vi "Sys A TXRX Host.vi"() -> ()   [LabVIEW 2019]
uses:
  SubVIs/mmWave HW Control/HW TXRX resources cluster.ctl
  <instrlib>/niMmWave/ni3610 and ni3630/controls/public/Board Information.ctl
  <instrlib>/niMmWave/ni3610 and ni3630/private/mm/Typedefs/PID.ctl
  <instrlib>/niMmWave/ni3610 and ni3630/controls/private/Board Hardware Revision.ctl
  SubVIs/mmWave HW Control/HW TXRX RF config cluster.ctl
  SubVIs/mmWave HW Control/HW Timing module config cluster.ctl
  SubVIs/mmWave HW Control/RX acquisition config.ctl
  SubVIs/Low-level/TypeDefs/TX trigger config.ctl
  FPGA/SubVIs/Utility/FPGA driver trigger source.ctl
  FPGA/SubVIs/Utility/FPGA driver trigger destination.ctl
  SubVIs/Low-level/TypeDefs/Front End Configuration.ctl
  SubVIs/Low-level/TypeDefs/Channel Configuration.ctl
  <instrlib>/niMmWave/ni3620/Config/v1/Host/Public/Typedefs/mmWave Port.ctl
  SubVIs/mmWave HW Control/HW state enum.ctl
  <vilib>/Utility/error.llb/DialogType.ctl
  SubVIs/mmWave HW Control/Message and Data cluster.ctl
  SubVIs/Low-level/TypeDefs/Hardware Configuration.ctl
  SubVIs/Low-level/TypeDefs/Direction.ctl
  SubVIs/Low-level/TypeDefs/Resources.ctl
  <vilib>/userdefined/High Color/nirio_resource_hc.ctl
  SubVIs/mmWave HW Control/TXRX generation acquisition config.ctl
  <vilib>/Analysis/4window.llb/windowTd.ctl
  <vilib>/measure/maspectr.llb/Power Spectrum and PSD Export Mode.ctl
  60642c00-3acc-4c81-b220-e8d2fc82becf.vi
  <vilib>/Analysis/2dsp.llb/1D Convolution (CDB).vi
  <vilib>/measure/maspectr.llb/FFT Power Spectrum and PSD for 1 Chan.vi
  Intertarget communication/NS master_class/NS master.lvclass
  SubVIs/mmWave HW Control/mmWave HW Control.lvlib
  <vilib>/Analysis/NI_AALPro.lvlib
  <instrlib>/niMmWave/ni3610 and ni3630/ni3610_and_ni3630_Driver_Lib.lvlib
  <instrlib>/niMmWave/ni3620/Config/v1/Host/niMmWave Config v1 Host.lvlib
  FPGA/SubVIs/Utility/FPGA Utility.lvlib
  <vilib>/measure/NI_MAPro.lvlib
  SubVIs/FPGA sequener API/FPGA sequencer API.lvlib
panel:
  out "burst memo":enum16{"DRAM", "BRAM"}(ring)
  out "last wr addr":u32
  in  "txrx.trigger":bool
  in  "stop scirpt":bool
  in  "Data view tab":T1(tab)
  out "Waveform plot":sgl[][](graph)
  in  "Averaging control":bool
  out "Power spectrum":cluster{"f0":dbl, "df":dbl, "magnitude":dbl[]}(graph)
  in  "averaging parameters":T2={"averaging mode"=enum."Peak hold", "weighting mode"=enum."Exponential", "number of averages"=50} {"number of averages" min=1}
  out "RXB-TXA stat":cluster{"Count":i32, "Mean":dbl, "Std":dbl} {"Std" format="%#_6p"; "Mean" format="%#_6p"}
  in  "Reset statistics":bool
  out "Time histogram":T3(graph) caption="XY Graph - Dark"
  out "RXA-TXA stat":cluster{"Count":i32, "Mean":dbl, "Std":dbl} {"Std" format="%#_6p"; "Mean" format="%#_6p"}
  out "RXB-RXA stat":cluster{"Count":i32, "Mean":dbl, "Std":dbl} {"Std" format="%#_6p"; "Mean" format="%#_6p"}
  in  "Repeat script":i32
  in  "Script.start":bool
  in  "Script":string="A \"hw.init\"\nB \"hw.reinit\" D 45000\nA \"txrx.start\" D500\nB \"rx.start\" D2000\nA \"txrx.trigger\" D200 R100\nA \"txrx.stop\"\nB \"rx.stop\""
  out "Last executed command":T4={"System"="", "Command"="", "Delay"=0, "Repeat"=1}
  out "script ctr":i32
  out "step ctr":i32
  out "R ctr":i32
  out "TX IQ":cdb[](array[numeric])
  out "Samples":u32
  out "coerced device configuration [channel]":T5[](array[typedef])=[{"port select"=enum."Loopback", "Rx hardware configuration"={"gain (dB)"=15.0, "frequency (Hz)"=12000000000.0, "mmWave adapter"="None", "adapter active port"=""}, "Tx hardware configuration"={"gain (dB)"=-15.0, "frequency (Hz)"=12000000000.0, "mmWave adapter"="None", "adapter active port"=""}}] {"Tx hardware configuration"."frequency (Hz)" format="%#_6p"; "Rx hardware configuration"."frequency (Hz)" format="%#_6p"}
  out "RXB-TX delay":dbl format="%#.3ps"
  out "Tx information":T8={"product code"=30638, "hardware revision"=enum."B", "serial number"="MTX1008\u0000"} {"product code" items=["PXIe-3610 I/Q Generator"=30638, "PXIe-3630 I/Q Digitizer"=30639]}
  in  "txrx.stop":bool
  out "Elements Remaining":u32
  in  "Stop Button":bool
  out "error out":T11
  in  "Tab Control":T12(tab)
  in  "HW.TXRX resources":T13={"TX_DAC"="Tx_DAC", "TX_FPGA"="Tx_FPGA", "IF"="IF_mod_demod", "RX_ADC"="Rx_ADC", "RX_FPGA"="Rx_FPGA"} caption="Reciever resources"
  in  "RF config":T14={"TX.Frequency"=0.0, "TX.Gain"=-10.0, "TX.mmWave adapter"="mmWave1/0", "RX.Frequency"=76000000000.0, "RX.Gain"=0.0, "RX.mmWave adapter"="mmWave0/0"} {"RX.Frequency" format="%#_6pHz"; "RX.Gain" format="%#_6fdb"; "TX.Frequency" format="%#_6pHz"; "TX.Gain" format="%#_6pHz"}
  in  "hw.init":bool
  in  "TX trigger options":T15
  in  "hw.conf trig":bool
  in  "HW.trig share config":T18={"mode"=enum."Export trig", "Timing module"="Dev1", "PXI line"="PXI_Trig1", "Module terminal"="PFI2"}
  in  "RX trigger options":T15={"delay"=8e-07, "trig source"=enum."Use Tclk", "PXI src"=0, "export"=enum."Synced trig", "PXI dest"=1} {"delay" format="%.0p"}
  in  "Repeat":bool
  in  "IQ waveform":string(combo)
  out "IQ preview":waveform(dbl)[](graph)
  out "Status":string
  in  "SysB.stop rx":bool
  in  "SysB.start rx":bool
  in  "SysB.hw reinit":bool
  in  "SysB.Connect":bool
  in  "Sys B IP address":string="192.168.40.171"
  in  "Plot":bool=TRUE
  out "dt":dbl=3.2552083333333335e-10 format="%#_6ps"
  in  "RX.read config":T19={"Samples"=320000}
  in  "txrx.start":bool
  out "Rx information":T8={"product code"=30639, "hardware revision"=enum."Unknown", "serial number"=""} {"product code" items=["PXIe-3610 I/Q Generator"=30638, "PXIe-3630 I/Q Digitizer"=30639]}
  out "RXA-TX delay":dbl format="%#.3ps"
  out "compensated max":i32
  out "max corr index":i32
  out "State":string
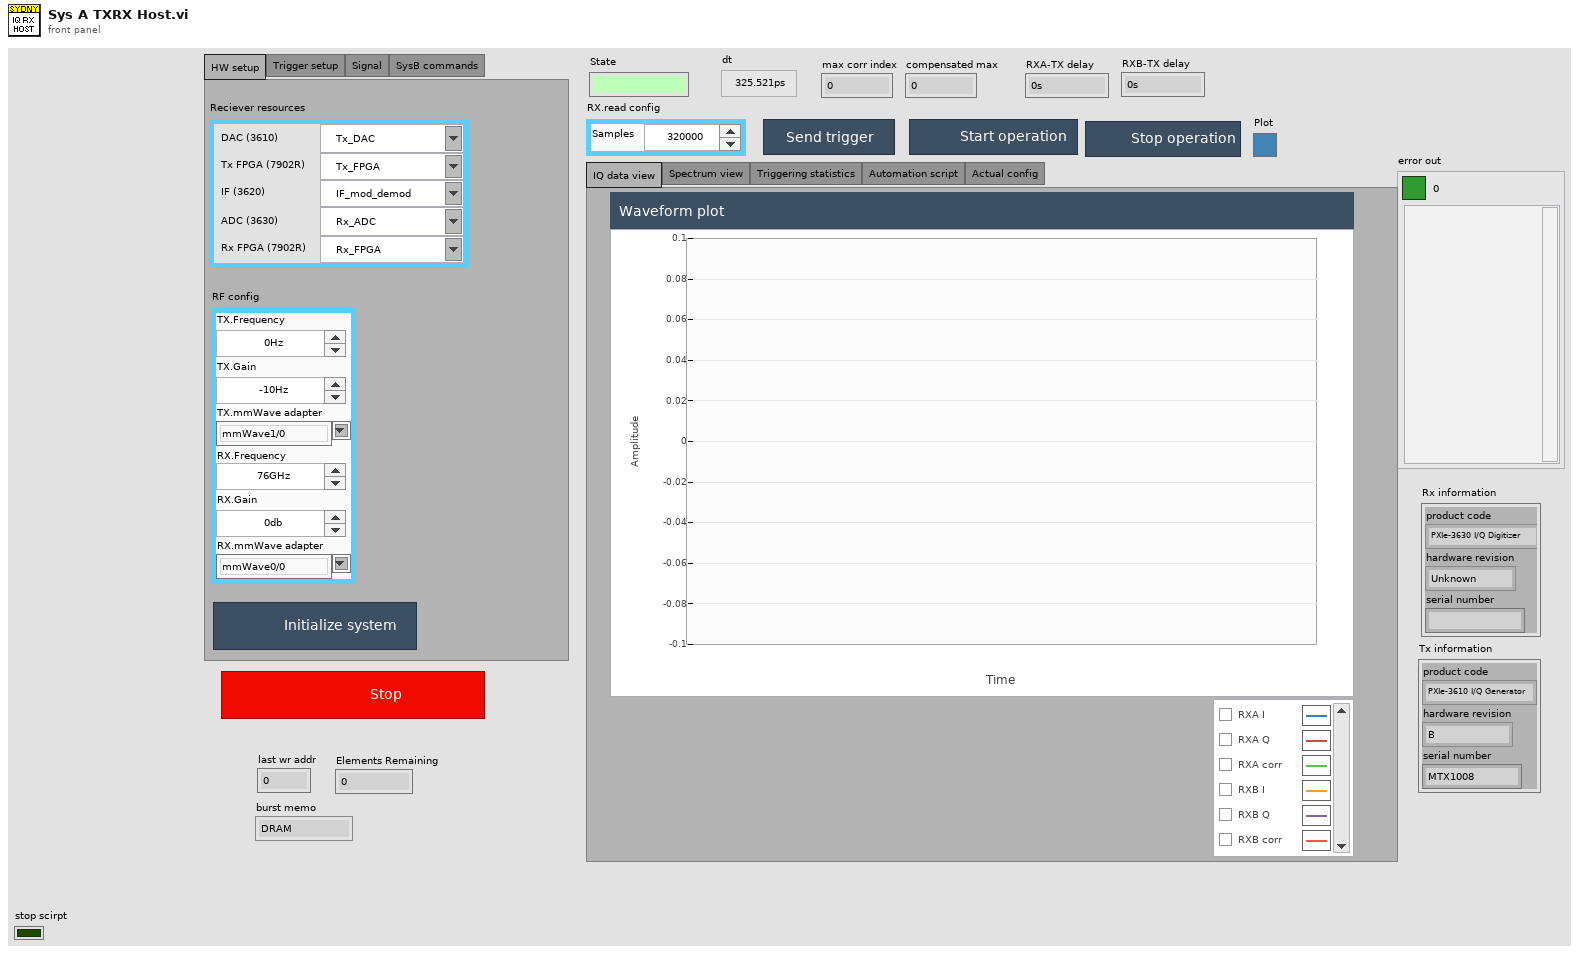
[diagram p1: front panel]
types:
  T1 = enum32{"IQ data view", "Spectrum view", "Triggering statistics", "Automation script", "Actual config"}
  T2 = cluster{"averaging mode":enum16{"No averaging", "Vector averaging", "RMS averaging", "Peak hold"}, "weighting mode":enum16{"Linear", "Exponential"}, "number of averages":u32}
  T3 = cluster{"X Values":dbl[], "Histogram: h(x)":i32[]}[]
  T4 = cluster{"System":string, "Command":string, "Delay":i32, "Repeat":i32}
  T5 = typedef "Front End Configuration.ctl" = cluster{"port select":enum16{"IF Port", "Loopback", "Sync Port"}, "Rx hardware configuration":T6, "Tx hardware configuration":T6}
  T6 = typedef "Channel Configuration.ctl" = cluster{"gain (dB)":dbl, "frequency (Hz)":dbl, "mmWave adapter":string, "adapter active port":T7}
  T7 = typedef "niMmWave Config v1 Host.lvlib/mmWave Port.ctl" = string
  T8 = typedef "Board Information.ctl" = cluster{"product code":T9, "hardware revision":T10, "serial number":string}
  T9 = typedef "ni3610_and_ni3630_Driver_Lib.lvlib/PID.ctl" = u16
  T10 = typedef "Board Hardware Revision.ctl" = enum16{"Unknown", "A", "B", "C", "D", "E", "F", "G", "H"}
  T11 = cluster{"Boolean Round":bool, "code":i32, "source":string}
  T12 = enum32{"HW setup", "Trigger setup", "Signal", "SysB commands"}
  T13 = typedef "mmWave HW Control.lvlib/HW TXRX resources cluster.ctl" = cluster{"TX_DAC":refnum<visa-resource-name>, "TX_FPGA":tag, "IF":tag, "RX_ADC":refnum<visa-resource-name>, "RX_FPGA":tag}
  T14 = typedef "mmWave HW Control.lvlib/HW TXRX RF config cluster.ctl" = cluster{"TX.Frequency":dbl, "TX.Gain":dbl, "TX.mmWave adapter":string, "RX.Frequency":dbl, "RX.Gain":dbl, "RX.mmWave adapter":string}
  T15 = typedef "TX trigger config.ctl" = cluster{"delay":dbl, "trig source":T16, "PXI src":i32, "export":T17, "PXI dest":i32}
  T16 = typedef "FPGA Utility.lvlib/FPGA driver trigger source.ctl" = enum16{"Use Tclk", "PXI_Trig", "Aurora RX trig"}
  T17 = typedef "FPGA Utility.lvlib/FPGA driver trigger destination.ctl" = enum16{"None", "Source trig", "Synced trig", "Delayed sync"}
  T18 = typedef "mmWave HW Control.lvlib/HW Timing module config cluster.ctl" = cluster{"mode":enum16{"None", "Export trig", "Import trig"}, "Timing module":tag, "PXI line":string, "Module terminal":string}
  T19 = typedef "mmWave HW Control.lvlib/RX acquisition config.ctl" = cluster{"Samples":u32}
  T20 = typedef "mmWave HW Control.lvlib/HW state enum.ctl" = enum16{"idle", "configuration", "running", "exit"}
  T21 = typedef "mmWave HW Control.lvlib/Message and Data cluster.ctl" = cluster{"message":string, "data":variant}
  T22 = typedef "Resources.ctl" = cluster{"7902R (Tx)":T23, "3610 (Tx)":refnum<visa-resource-name>, "3620 (IF)":T23, "3630 (RX)":refnum<visa-resource-name>, "7902R (Rx)":T23}
  T23 = typedef "nirio_resource_hc.ctl" = tag
  T24 = typedef "mmWave HW Control.lvlib/TXRX generation acquisition config.ctl" = cluster{"RX.read config":T19, "TX.IQ signal":cdb[], "TX.IQ Fs":dbl, "TX burst/continuous":bool, "TX.IQ samples":i32}
  T25 = typedef "Direction.ctl" = enum16{"Transceiver", "Receiver", "Transmitter"}
  T26 = cluster{"start addr":u32, "end addr":u32, "repeat":u64}
  T27 = typedef "DialogType.ctl" = u16
  T28 = typedef "Hardware Configuration.ctl" = cluster{"direction":T25, "baseband only":bool}
  T29 = typedef "Session.ctl" = cluster{"3620 session":refnum<queue>, "tx baseband session":T30, "rx baseband session":T38, "tx gain (dB)":dbl, "rx gain (dB)":dbl, "hardware configuration":T28, "gain ranging":T39[], "pxi trigger bus information":T40}
  T30 = typedef "Tx Baseband Session.ctl" = cluster{"3610 session":T31, "7902 reference":T37}
  T31 = typedef "ni3610_and_ni3630_Driver_Lib.lvlib/Main Settings.ctl" = cluster{"VISA resource name":refnum<visa-resource-name>, "Address Space":T32, "window_offset":u32, "register_addresses":T33, "required_MM_fpga_version":cluster{"signature":u32, "hardware":u32, "current revision":u32, "oldest revision":u32}, "CPLD Oldest Compat Version ":cluster{"hardware":u32, "CPLD firmware":u32}, "MM_FPGA_image_location":string, "is_init":bool, "card_type":T34, "DacLmkConfigFileName":string, "AdcLmkConfigFileName":string, "AdcConfigFileName":string, "DacConfigFileName_RevA":string, "DacConfigFileName_RevB":string, "Mulde hardware revision":u8, "bypass DAC PLL\n":bool, "IQ Card Revision":T35, "board capability":T36}
  T32 = typedef "VISA Register Access Address Space.ctl" = u16
  T33 = typedef "ni3610_and_ni3630_Driver_Lib.lvlib/Register Adresses.ctl" = cluster{"MM based Registers":cluster{"Revision":u32, "OldestCompatRev":u32, "signature":u32, "scratch":u32, "LedControl":u32, "BoardHwRev":u32, "BoardControl":u32, "ThermalStatus":u32, "BasebandStatus":u32, "BasebandControl":u32, "BasebandAuxSetup":u32, "BasebandAuxStatus":u32, "LmkSyncOutSetup":u32, " AdcSyncOutSetup":u32, " InjSyncOutSetup":u32, " PxiTrig0OutSetup":u32, " PxiTrig1OutSetup":u32, " PxiTrig2OutSetup":u32, " PxiTrig3OutSetup":u32, " PxiTrig4OutSetup":u32, " PxiTrig5OutSetup":u32, " PxiTrig6OutSetup":u32, " PxiTrig7OutSetup":u32}, "CPLD based Registers":cluster{"SlaveSignature":u32, "SlaveRevision":u32, "SlaveOldestCompatRev":u32, "SlaveScratch":u32, "SlaveSetup":u32, "SlaveStatus":u32, "IDacReg_offset":u32, "LMKRegGrp0_offset":u32, "QDacReg_offset":u32, "BrdTempSensorVal":u32, "TempSensorPowerDown":u32, "GPIOReg_offset":u32, "IAdcReg_offset":u32, "QAdcReg_offset":u32, "LMKRegGrp1_offset":u32, "QadcTempSensorVal":u32, "IadcTempSensorVal":u32, "RevisionReg":u32, "VcxoReg":u32, "CpldStatusReg":u32, "PowerReg":u32, "VBiasEnReg":u32, "ExtRefOeReg":u32, "QdacCtrlReg":u32, "QdacStatusReg":u32, "IdacCtrlReg":u32, "IdacStatusReg":u32, "QdacJtagIn":u32, "QdacJtagOut":u32, "IdacJtagIn":u32, "IdacJtagOut":u32, "IqDcSetupReg":u32, "QadcStatusReg":u32, "IadcStatusReg":u32, "BrdSetupReg":u32, "IqDcRevisionReg":u32, "PllStatusReg":u32, "EndpointScratchReg":u32, "AdcSyncCfgReg":u32, "IqCardOpampReg":u32}, "CPLD Register Offset":u32, "MM  Register Offset":u32, " PxiTrig0OutSetup":u32}
  T34 = typedef "ni3610_and_ni3630_Driver_Lib.lvlib/Base Card Type.ctl" = enum16{"unspecified", "ADC", "DAC"}
  T35 = typedef "ni3610_and_ni3630_Driver_Lib.lvlib/IQ Card Revision.ctl" = enum16{"RevA", "RevB", "RevC", "RevD"}
  T36 = typedef "ni3610_and_ni3630_Driver_Lib.lvlib/Board Capability.ctl" = cluster{"baseband sync":enum16{"no baseband sync", "baseband sync"}}
  T37 = typedef "Blank FPGA Reference.ctl" = refnum<k20>
  T38 = typedef "Rx Baseband Session.ctl" = cluster{"3630 session":T31, "7902 reference":T37}
  T39 = typedef "Gain Ranging.ctl" = cluster{"gain ranging active scope":string, "gain ranging stream session":refnum<k20>}
  T40 = typedef "PXI Trigger Bus Info.ctl" = cluster{"chassis resource name":refnum<visa-resource-name>, "7902R (TX)":i16, "3610 (TX)":i16, "3620 (IF)":i16, "3630 (RX)":i16, "7902R (RX)":i16}
  T41 = typedef "Constants.ctl" = cluster{"data clock rate (Hz)":dbl, "sample rate (Hz)":dbl, "sample rate selector string":string, "default tx bitfile path":path, "default rx bitfile path":path, "default proc bitfile path":path}
  T42 = typedef "NI_MAPro.lvlib/Power Spectrum and PSD Export Mode.ctl" = u16
  T43 = typedef "NI_AALPro.lvlib/windowTd.ctl" = u32
  T44 = cluster{"X Values":dbl[], "Histogram: h(x)":i32[]}
  T45 = typedef "FPGA sequencer API.lvlib/FPGA sequencer ref.ctl" = refnum<k20>
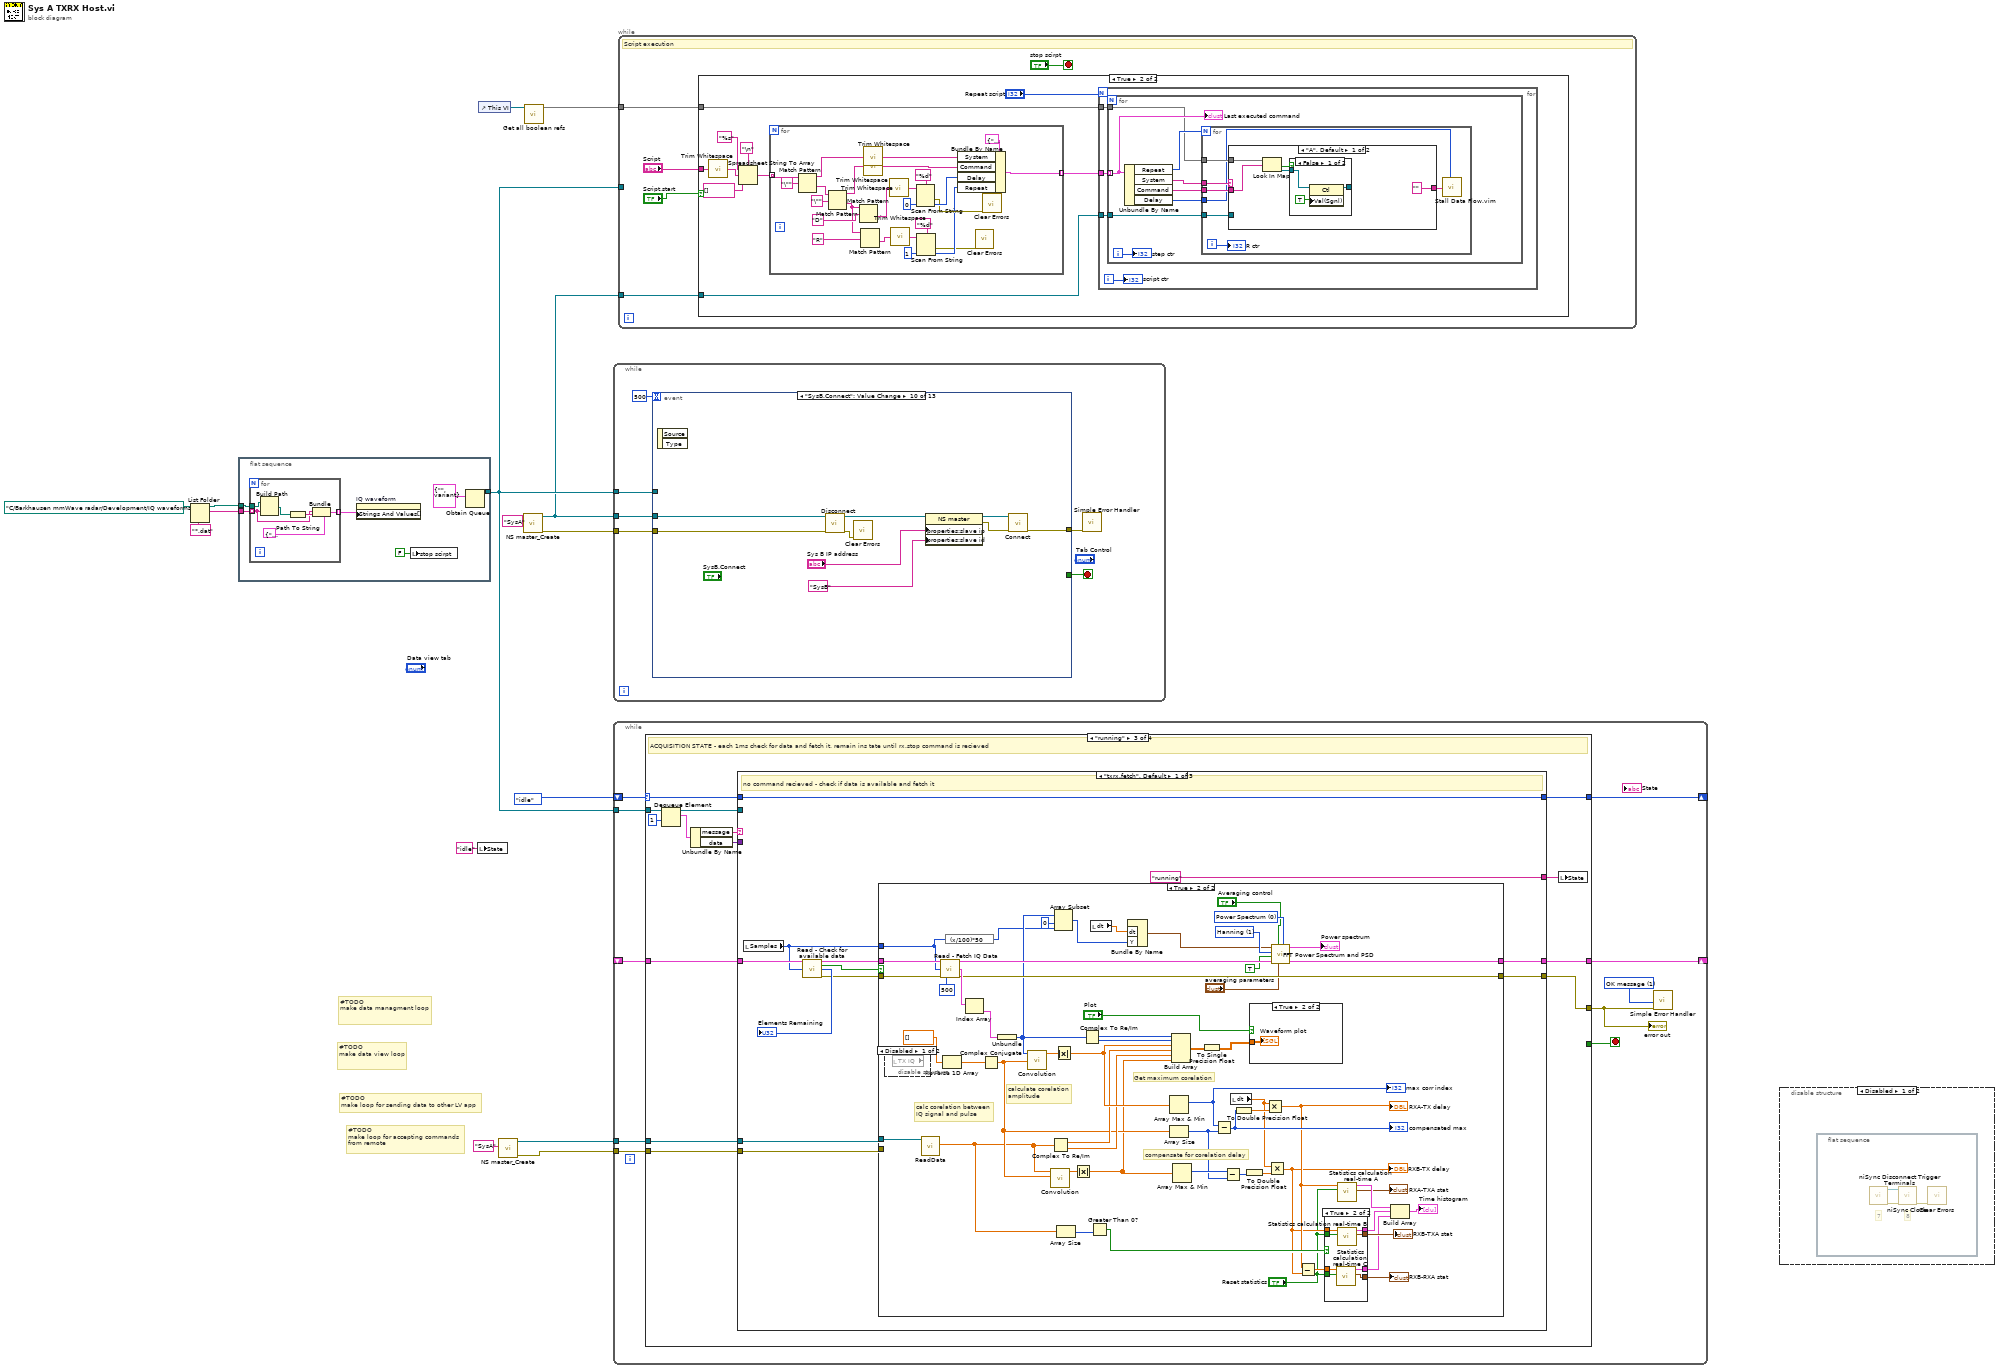
[diagram p0: block diagram]
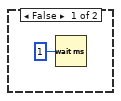
[diagram p2: hidden frame]
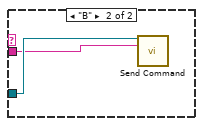
[diagram p4: hidden frame]
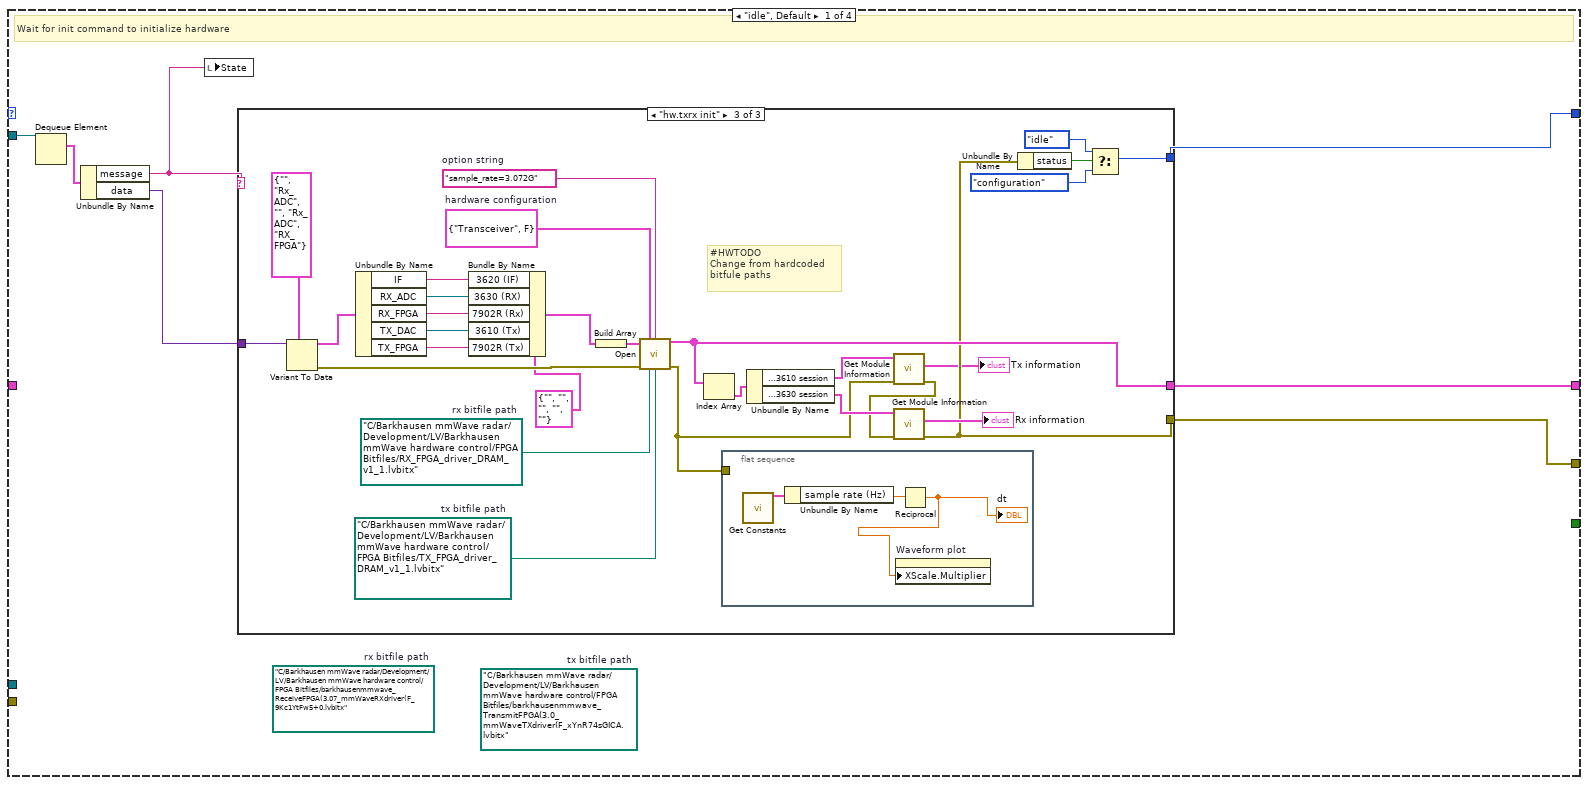
[diagram p6: hidden frame]
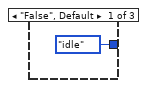
[diagram p7: hidden frame]
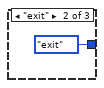
[diagram p8: hidden frame]
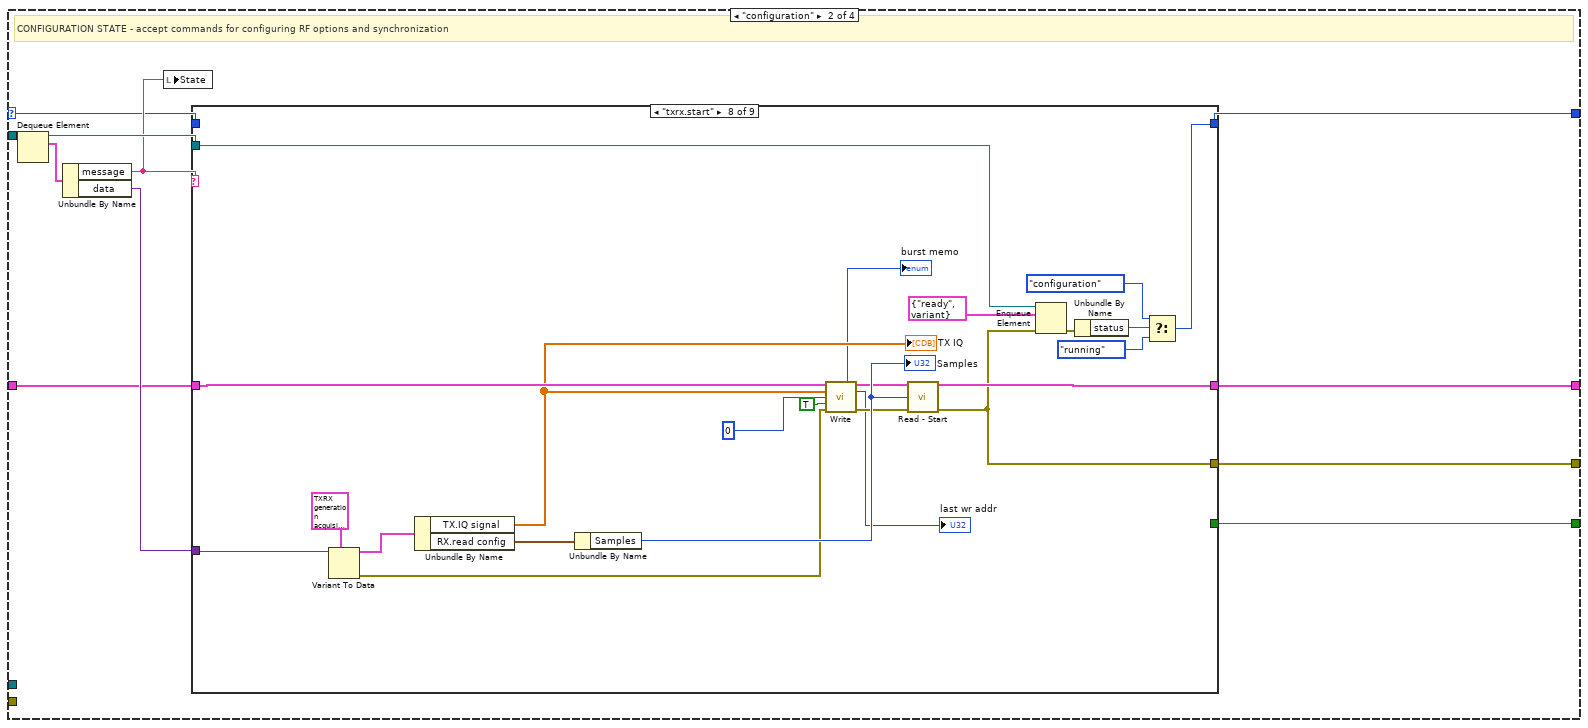
[diagram p9: hidden frame]
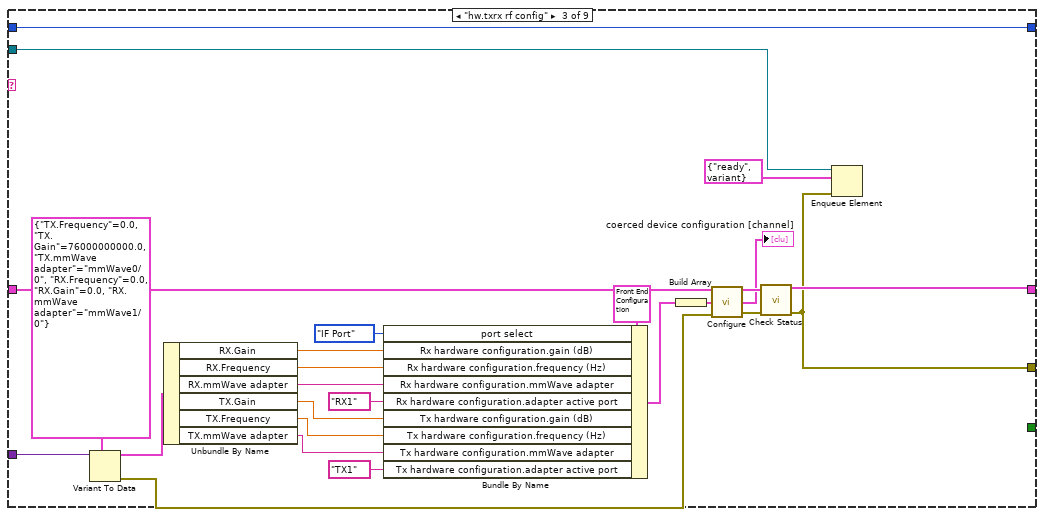
[diagram p12: hidden frame]
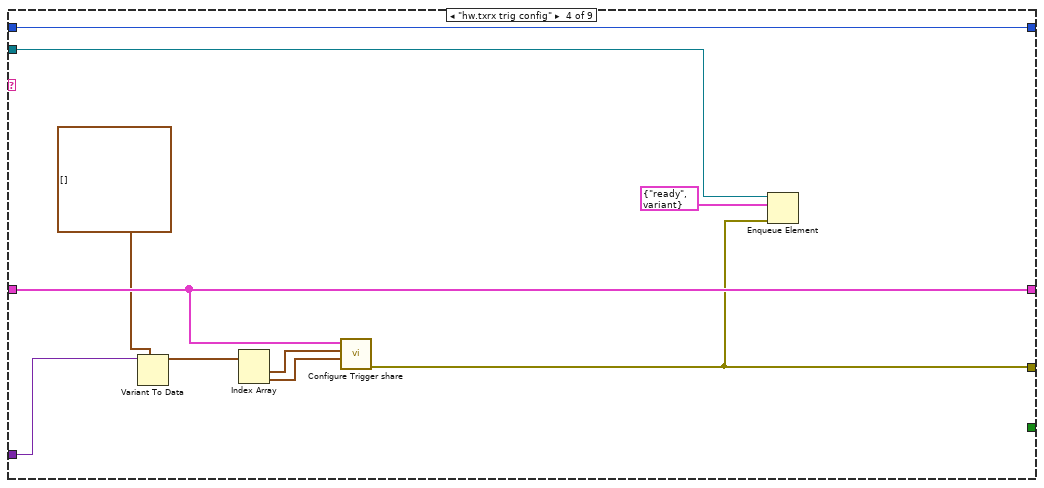
[diagram p13: hidden frame]
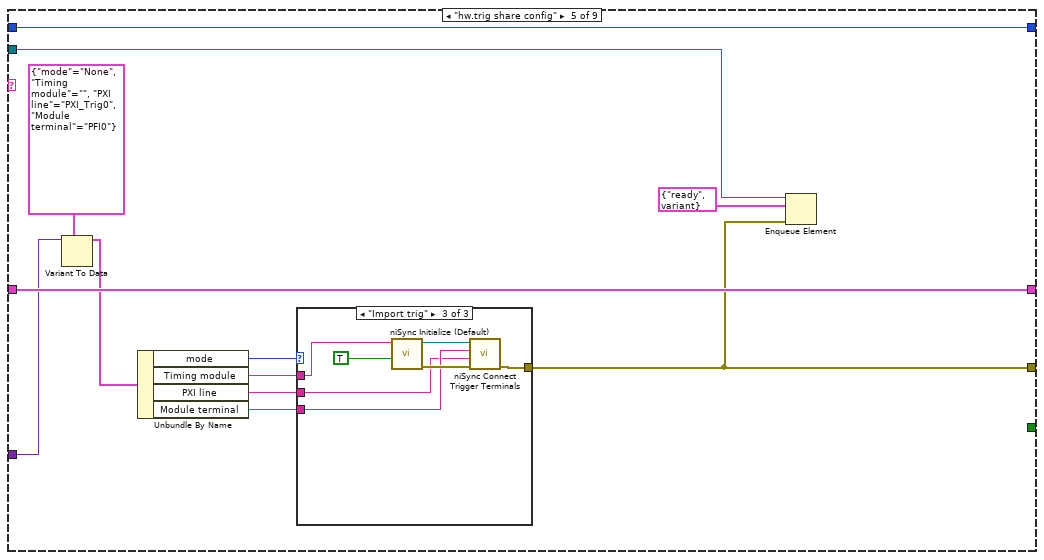
[diagram p14: hidden frame]
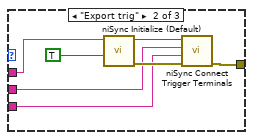
[diagram p16: hidden frame]
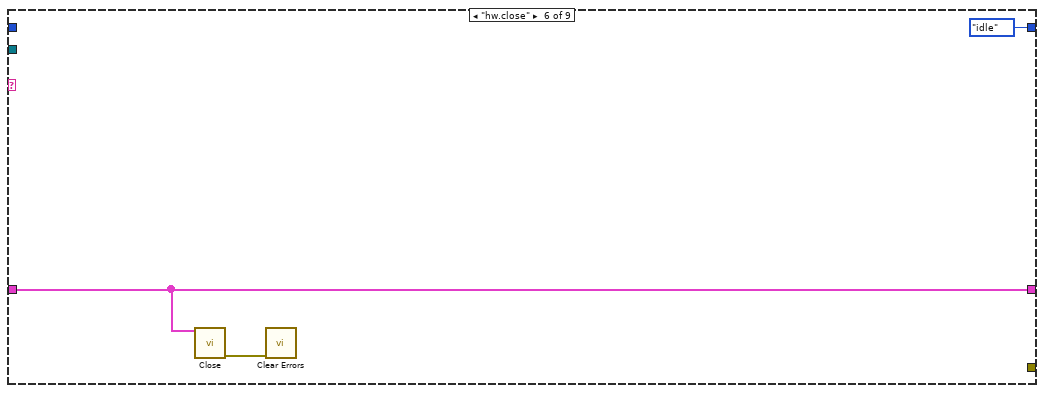
[diagram p17: hidden frame]
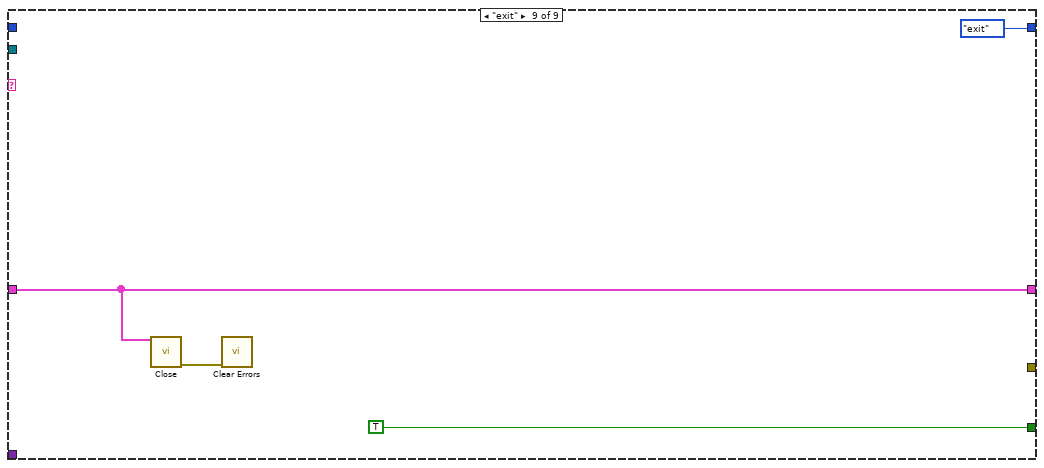
[diagram p19: hidden frame]
diagram:
  # "#TODO\nmake loop for sending data to other LV app"
  # "#TODO\nmake loop for accepting commands\nfrom remote"
  # "#TODO\nmake data view loop"
  # "#TODO\nmake data managment loop"
  n1 = List Folder(path=path "C:/Barkhausen mmWave radar/Development/IQ waveforms" ("IQ waveform (.dat) 2"), pattern="*.dat") -> (path out=w1:path, filenames=w2:string[])  [unwired: 2 in, 2 out]
  n2 = flat-sequence {
    tunnel: [w20] -> w8
    tunnel: w2 -> [w18]
    tunnel: w1 -> [w17]
    frame #0 {
      n3 = for {
        tunnel: w18 -> [w23] mode=indexing
        tunnel: w17 -> [w27]
        tunnel: [w22] -> w16 mode=indexing
        n4 = Build Path(base path=w27, name or relative path=w23) -> (appended path=w25:path)
        n5 = Path To String(path=w25) -> (string=w24:string)
        n6 = Bundle(cluster=cluster{"String":string, "Value":string} {"String"="", "Value"=""}, "String"=w23, "Value"=w24) -> (w22:cluster{"String":string, "Value":string})
      }
      n7 = property on="IQ waveform" class="CmbBox"("Strings And Values[]"=w16) -> ()  [unwired: 2 in, 2 out]
      n8 = local write "stop scirpt"(FALSE ("stop scirpt")) -> ()
      n9 = Obtain Queue(element data type=T21 {"message"="", "data"=variant} ("Message data cluster")) -> (queue out=w20:refnum<queue>)  [unwired: 4 in, 2 out]
    }
  }
  n10 = local write "State"("idle" ("State")) -> ()
  n11 = control-ref of="This VI"() -> (w7:refnum<vi>)
  n12 = call "NS master_Create.vi"("ID"="SysA") -> ("error out"=w11:errorcluster, "reference out"=w12:refnum<class "NS master.lvclass">)  [unwired: 9 in]
  n13 = call "NS master_Create.vi"("ID"="SysA") -> ("error out"=w9:errorcluster, "reference out"=w5:refnum<class "NS master.lvclass">)  [unwired: 9 in]
  n14 = call "Get all boolean refs.vi"("VI"=w7) -> ("Boolean ref map"=w6:map{string, refnum<vi>})  [unwired: 10 in]
  n15 = while {
    tunnel: w8 -> [w33]
    shift-right: [w36] -> _
    shift-left: _ -> [w35]
    shift-right: [w30] -> _
    shift-left: HW_state_enum."idle" ("hw state") -> [w31]
    tunnel: w11 -> [w29]
    tunnel: w12 -> [w28]
    stop <- w37 stop-if-true
    w32 = T27 1 items=["no dialog", "OK message", "continue or stop message", "OK message + warnings", "continue/stop + warnings"] ("type of dialog (OK msg:1)")
    n16 = case shown="\"running\"" w31 {
      selector: w31 -> [_ w80 w197 w315]
      tunnel: [_ w88 _ TRUE] -> w37
      tunnel: [w40 w86 w192 w314] -> w36
      tunnel: w35 -> [_ w85 w193 w314]
      tunnel: [w38 w84 w191 _] -> w34
      tunnel: w33 -> [w43 w83 w199 _]
      tunnel: [w39 w79 w194 w315] -> w30
      tunnel: w29 -> [_ _ w188 _]
      tunnel: w28 -> [_ _ w187 _]
      frame "idle", Default {
        (unwired) path "C:/Barkhausen mmWave radar/Development/LV/Barkhausen mmWave hardware control/FPGA Bitfiles/barkhausenmmwave_TransmitFPGA(3.0_mmWaveTXdriver(F_xYnR74sGICA.lvbitx"  # tx bitfile path
        (unwired) path "C:/Barkhausen mmWave radar/Development/LV/Barkhausen mmWave hardware control/FPGA Bitfiles/barkhausenmmwave_ReceiveFPGA(3.07_mmWaveRXdriver(F_9Kc1YtFw5+0.lvbitx"  # rx bitfile path
        # "Wait for init command to initialize hardware"
        n17 = Dequeue Element(queue=w43) -> (element=w44:T21)  [unwired: 2 in, 3 out]
        n18 = Unbundle By Name(w44) -> ("message"=w42:string, "data"=w41:variant)
        n19 = local write "State"(w42) -> ()
        n20 = case shown="\"hw.txrx init\"" w42 {
          tunnel: w41 -> [_ _ w59]
          tunnel: [_ _ w58] -> w40
          tunnel: [HW_state_enum."idle" ("hw state") HW_state_enum."exit" ("hw state") w54] -> w39
          tunnel: [_ _ w53] -> w38
          frame "False", Default {
          }
          frame "exit" {
          }
          frame "hw.txrx init" {
            w63 = "sample_rate=3.072G"  # option string
            w62 = path "C:/Barkhausen mmWave radar/Development/LV/Barkhausen mmWave hardware control/FPGA Bitfiles/RX_FPGA_driver_DRAM_v1_1.lvbitx"  # rx bitfile path
            w61 = path "C:/Barkhausen mmWave radar/Development/LV/Barkhausen mmWave hardware control/FPGA Bitfiles/TX_FPGA_driver_DRAM_v1_1.lvbitx"  # tx bitfile path
            w74 = T28 {"direction"=enum."Transceiver", "baseband only"=FALSE}  # hardware configuration
            # "#HWTODO\nChange from hardcoded\nbitfule paths"
            n21 = Variant To Data(type=T13 {"TX_DAC"="", "TX_FPGA"="Rx_ADC", "IF"="", "RX_ADC"="Rx_ADC", "RX_FPGA"="RX_FPGA"} ("HW.RX resources"), Variant=w59) -> (data=w75:T13, error out=w65:errorcluster)  [unwired: 1 in]
            n22 = Unbundle By Name(w75) -> ("IF"=w71:tag, "RX_ADC"=w70:refnum<visa-resource-name>, "RX_FPGA"=w69:tag, "TX_DAC"=w52:refnum<visa-resource-name>, "TX_FPGA"=w51:tag)
            n23 = Bundle By Name(cluster=T22 {"7902R (Tx)"="", "3610 (Tx)"="", "3620 (IF)"="", "3630 (RX)"="", "7902R (Rx)"=""} ("resources"), "3620 (IF)"=w71, "3630 (RX)"=w70, "7902R (Rx)"=w69, "3610 (Tx)"=w52, "7902R (Tx)"=w51) -> (w73:T22)
            n24 = Build Array(w73) -> (w72:T22[])
            n25 = call "Open.vi"("resources"=w72, "hardware configuration"=w74, "option string"=w63, "error in"=w65, "rx bitfile path"=w62, "tx bitfile path"=w61) -> ("session out"=w58:T29[], "error out"=w49:errorcluster)  [unwired: 7 in, 1 out]
            n26 = Index Array(array=w58) -> (element=w68:T29)  [unwired: 1 in]
            n27 = flat-sequence {
              tunnel: w49 -> [_]
              frame #0 {
                n28 = call "Get Constants.vi"() -> ("constants"=w78:T41)  [unwired: 15 in]
                n29 = Unbundle By Name(w78) -> ("sample rate (Hz)"=w77:dbl)
                n30 = Reciprocal(x=w77) -> (1/x=w76:dbl)
                "dt" <- w76
                n31 = property on="Waveform plot" class="WFGraph (strict)"("XScale.Multiplier"=w76) -> ()  [unwired: 2 in, 2 out]
              }
            }
            n32 = Unbundle By Name(w68) -> ("tx baseband session.3610 session"=w50:T31, "rx baseband session.3630 session"=w67:T31)
            n33 = call <instrlib>:"Get Module Information.vi"("error in (no error)"=w49, "Board Settings in"=w50) -> ("error out"=w48:errorcluster, "board information"=→"Tx information":T8)  [unwired: 7 in, 1 out]
            n34 = call <instrlib>:"Get Module Information.vi"("error in (no error)"=w48, "Board Settings in"=w67) -> ("error out"=w53:errorcluster, "board information"=→"Rx information":T8)  [unwired: 7 in, 1 out]
            n35 = Unbundle By Name(w53) -> ("status"=w57:bool)
            n36 = Select(t=HW_state_enum."idle" ("hw state"), s=w57, f=HW_state_enum."configuration" ("hw state")) -> (s? t:f=w54:T20)
          }
        }
      }
      frame "configuration" {
        # "CONFIGURATION STATE - accept commands for configuring RF options and synchronization"
        n37 = Dequeue Element(queue=w83) -> (queue out=w82:refnum<queue>, element=w89:T21)  [unwired: 2 in, 2 out]
        n38 = Unbundle By Name(w89) -> ("message"=w81:string, "data"=w87:variant)
        n39 = local write "State"(w81) -> ()
        n40 = case shown="\"txrx.start\"" w81 {
          tunnel: [_ _ _ _ _ _ _ _ TRUE] -> w88
          tunnel: w87 -> [_ _ w118 w128 w139 _ _ w182 _]
          tunnel: [w91 w93 w105 w127 w140 w156 w159 w173 w185] -> w86
          tunnel: w85 -> [w91 w93 w116 w127 w140 w156 w159 w168 w185]
          tunnel: [_ _ w101 w123 w130 _ _ w172 _] -> w84
          tunnel: w82 -> [_ _ w102 w124 w131 _ _ w181 _]
          tunnel: w80 -> [w90 w92 w100 w122 w129 _ w158 _ _]
          tunnel: [w90 w92 w100 w122 w129 HW_state_enum."idle" ("hw state") w158 w175 HW_state_enum."exit" ("hw state")] -> w79
          frame Default {
          }
          frame "----HARDWARE CONFIG----" {
          }
          frame "hw.txrx rf config" {
            n41 = Variant To Data(type=T14 {"TX.Frequency"=0.0, "TX.Gain"=76000000000.0, "TX.mmWave adapter"="mmWave0/0", "RX.Frequency"=0.0, "RX.Gain"=0.0, "RX.mmWave adapter"="mmWave1/0"} ("TXRX config"), Variant=w118) -> (data=w115:T14, error out=w104:errorcluster)  [unwired: 1 in]
            n42 = Unbundle By Name(w115) -> ("RX.Gain"=w108:dbl, "RX.Frequency"=w109:dbl, "RX.mmWave adapter"=w110:string, "TX.Gain"=w99:dbl, "TX.Frequency"=w98:dbl, "TX.mmWave adapter"=w97:string)
            n43 = Bundle By Name(cluster=T5 {"port select"=enum."Loopback", "Rx hardware configuration"={"gain (dB)"=15.0, "frequency (Hz)"=12000000000.0, "mmWave adapter"="None", "adapter active port"=""}, "Tx hardware configuration"={"gain (dB)"=-15.0, "frequency (Hz)"=12000000000.0, "mmWave adapter"="None", "adapter active port"=""}} ("device configuration [channel]"), "port select"=enum16{"IF Port", "Loopback", "Sync Port"}."IF Port", "Rx hardware configuration.gain (dB)"=w108, "Rx hardware configuration.frequency (Hz)"=w109, "Rx hardware configuration.mmWave adapter"=w110, "Rx hardware configuration.adapter active port"=T7 "RX1", "Tx hardware configuration.gain (dB)"=w99, "Tx hardware configuration.frequency (Hz)"=w98, "Tx hardware configuration.mmWave adapter"=w97, "Tx hardware configuration.adapter active port"=T7 "TX1") -> (w112:T5)
            n44 = Build Array(w112) -> (w111:T5[])
            n45 = call "Configure.vi"("session in"=w116, "device configuration [channel]"=w111, "error in"=w104) -> ("session out"=w107:T29[], "coerced device configuration [channel]"=→"coerced device configuration [channel]":T5[], "error out"=w106:errorcluster)  [unwired: 10 in]
            n46 = call "Check Status.vi"("session in"=w107, "error in"=w106) -> ("session out"=w105:T29[], "error out"=w101:errorcluster)  [unwired: 9 in, 3 out]
            n47 = Enqueue Element(queue=w102, element=T21 {"message"="ready", "data"=variant}, error in (no error)=w101) -> ()  [unwired: 1 in, 3 out]
          }
          frame "hw.txrx trig config" {
            n48 = Variant To Data(type=T15[] [], Variant=w128) -> (data=w126:T15[])  [unwired: 1 in, 1 out]
            n49 = Index Array(array=w126) -> (element #1=w120:T15, element #2=w119:T15)  [unwired: 2 in]
            n50 = call "Configure Trigger share.vi"("RX trigger options"=w119, "TX trigger options"=w120, "session in"=w127) -> ("error out"=w123:errorcluster)  [unwired: 5 in, 3 out]
            n51 = Enqueue Element(queue=w124, element=T21 {"message"="ready", "data"=variant}, error in (no error)=w123) -> ()  [unwired: 1 in, 3 out]
          }
          frame "hw.trig share config" {
            n52 = Variant To Data(type=T18 {"mode"=enum."None", "Timing module"="", "PXI line"="PXI_Trig0", "Module terminal"="PFI0"} ("HW.trig share config"), Variant=w139) -> (data=w137:T18)  [unwired: 1 in, 1 out]
            n53 = Unbundle By Name(w137) -> ("mode"=w136:enum16{"None", "Export trig", "Import trig"}, "Timing module"=w135:tag, "PXI line"=w134:string, "Module terminal"=w133:string)
            n54 = case shown="\"Import trig\"" w136 {
              tunnel: w135 -> [_ w144 w151]
              tunnel: [_ w143 w150] -> w130
              tunnel: w134 -> [_ w142 w148]
              tunnel: w133 -> [_ w141 w149]
              frame "None", Default {
              }
              frame "Export trig" {
                n55 = call <instrlib>:"niSync Initialize (Default).vi"("reset device (F)"=TRUE ("reset device (False)"), "resource name"=w144) -> ("error out"=w147:errorcluster, "instrument handle out"=w146:refnum<k15>)  [unwired: 8 in]
                n56 = call <instrlib>:"niSync Connect Trigger Terminals.vi"("error in (no error)"=w147, "destination terminal"=w141, "source terminal"=w142, "instrument handle"=w146) -> ("error out"=w143:errorcluster)  [unwired: 6 in, 1 out]
              }
              frame "Import trig" {
                n57 = call <instrlib>:"niSync Initialize (Default).vi"("reset device (F)"=TRUE ("reset device (False)"), "resource name"=w151) -> ("error out"=w154:errorcluster, "instrument handle out"=w153:refnum<k15>)  [unwired: 8 in]
                n58 = call <instrlib>:"niSync Connect Trigger Terminals.vi"("error in (no error)"=w154, "destination terminal"=w148, "source terminal"=w149, "instrument handle"=w153) -> ("error out"=w150:errorcluster)  [unwired: 6 in, 1 out]
              }
            }
            n59 = Enqueue Element(queue=w131, element=T21 {"message"="ready", "data"=variant}, error in (no error)=w130) -> ()  [unwired: 1 in, 3 out]
          }
          frame "hw.close" {
            n60 = call "Close.vi"("session"=w156) -> ("error out"=w157:errorcluster)  [unwired: 14 in]
            n61 = call <vilib>:"Clear Errors.vi"("error in (no error)"=w157) -> ()  [unwired: 5 in, 2 out]
          }
          frame "----OPERATE----" {
          }
          frame "txrx.start" {
            n62 = Variant To Data(type=T24 {"RX.read config"={"Samples"=16000}, "TX.IQ signal"=[1.0+0.0i], "TX.IQ Fs"=50000000.0, "TX burst/continuous"=TRUE, "TX.IQ samples"=1600} ("TXRX config"), Variant=w182) -> (data=w170:T24, error out=w164:errorcluster)  [unwired: 1 in]
            n63 = Unbundle By Name(w170) -> ("TX.IQ signal"=w163:cdb[], "RX.read config"=w169:T19)
            "TX IQ" <- w163
            n64 = Unbundle By Name(w169) -> ("Samples"=w174:u32)
            "Samples" <- w174
            n65 = call "Write.vi"("session in"=w168, "data"=w163, "Wfm addr"=u32 0, "zero pad"=TRUE, "error in"=w164) -> ("burst memo"=→"burst memo":enum16{"DRAM", "BRAM"}, "session out"=w166:T29[], "last wr addr"=→"last wr addr":u32, "error out"=w165:errorcluster)  [unwired: 7 in]
            n66 = call "Read - Start.vi"("session in"=w166, "number of samples"=w174, "error in"=w165) -> ("session out"=w173:T29[], "error out"=w172:errorcluster)  [unwired: 11 in]
            n67 = Enqueue Element(queue=w181, element=T21 {"message"="ready", "data"=variant}, error in (no error)=w172) -> (error out=w176:errorcluster)  [unwired: 1 in, 2 out]
            n68 = Unbundle By Name(w176) -> ("status"=w179:bool)
            n69 = Select(t=HW_state_enum."configuration" ("hw state"), s=w179, f=HW_state_enum."running" ("hw state")) -> (s? t:f=w175:T20)
          }
          frame "exit" {
            n70 = call "Close.vi"("session"=w185) -> ("error out"=w184:errorcluster)  [unwired: 14 in]
            n71 = call <vilib>:"Clear Errors.vi"("error in (no error)"=w184) -> ()  [unwired: 5 in, 2 out]
          }
        }
      }
      frame "running" {
        # "ACQUISITION STATE - each 1ms check for data and fetch it. remain ins tate until rx.stop command is recieved"
        n72 = Dequeue Element(queue=w199, timeout in ms (-1)=1) -> (queue out=w189:refnum<queue>, element=w200:T21)  [unwired: 1 in, 2 out]
        n73 = Unbundle By Name(w200) -> ("message"=w196:string, "data"=w195:variant)
        n74 = case shown="\"txrx.fetch\", Default" w196 {
          tunnel: w197 -> [w212 w291 _]
          tunnel: w195 -> [_ _ _]
          tunnel: [w212 w291 HW_state_enum."configuration" ("hw state")] -> w194
          tunnel: w193 -> [w209 w284 w312]
          tunnel: [w211 w289 w312] -> w192
          tunnel: [w210 w283 _] -> w191
          tunnel: ["running" ("State") "trigger sent" ("State") "configuration" ("State")] -> w190
          tunnel: w189 -> [_ w288 _]
          tunnel: w188 -> [w202 _ _]
          tunnel: w187 -> [w201 _ _]
          frame "txrx.fetch", Default {
            # "no command recieved - check if data is available and fetch it"
            n75 = local read "Samples"() -> (w208:u32)
            n76 = call "Read - Check for available data.vi"("session in"=w209, "number of samples"=w208) -> ("session out"=w205:T29[], "data available"=w207:bool, "Elements Remaining"=→"Elements Remaining":u32, "error out"=w204:errorcluster)  [unwired: 10 in]
            n77 = case shown="True" w207 {
              tunnel: [w214 w260] -> w211
              tunnel: [w213 w258] -> w210
              tunnel: w208 -> [_ w220]
              tunnel: w205 -> [w214 w256]
              tunnel: w204 -> [w213 w255]
              tunnel: w202 -> [_ _]
              tunnel: w201 -> [_ w254]
              frame False {
              }
              frame True {
                w226 = T42 0 items=["Power Spectrum", "Power Spectral Density"] ("export mode")
                w228 = T43 1 items=["Rectangle"=0, "Hanning"=1, "Hamming"=2, "Blackman-Harris"=3, "Exact Blackman"=4, "Blackman"=5, "Flat Top"=6, "4 Term B-Harris "=7, "7 Term B-Harris"=8, "Low Sidelobe"=9, "Blackman Nuttall"=11, "Triangle"=30, "Bartlett-Hanning"=31, "Bohman"=32, "Parzen"=33, "Welch"=34, "Kaiser"=60, "Dolph-Chebyshev"=61, "Gaussian"=62] ("window")
                # "compensate for corelation delay"
                # "Get maximum corelation"
                # "calculate corelation\namplitude"
                # "calc corelation between \nIQ signal and pulse"
                n78 = disable-structure shown="Disabled" {
                  frame Disabled {
                    n79 = local read "TX IQ"() -> ()  [unwired: 1 out]
                  }
                  frame Enabled {
                  }
                }
                n80 = call-dynamic "ReadData.vi"("reference in"=w254) -> ("data"=w239:cdb[])  [unwired: 7 in, 3 out]
                n81 = call "Read - Fetch IQ Data.vi"("session in"=w256, "number of samples"=w220, "error in"=w255, "Timeout (ms)"=500) -> ("session out"=w260:T29[], "data [channel]"=w259:cluster{"data":i16[]}[], "error out"=w258:errorcluster)  [unwired: 9 in]
                n82 = Reverse 1D Array(array=dbl[] []) -> (reversed array=w265:dbl[])
                n83 = expression code="(x/100)*50"(w220) -> (w219:u32)
                n84 = Index Array(array=w259) -> (element=w270:cluster{"data":i16[]})  [unwired: 1 in]
                n85 = Complex Conjugate(1:w265) -> (0:w251:cdb[])
                n86 = Unbundle(w270) -> ("data"=w222:i16[])
                n87 = call-poly <vilib>:"Convolution.vi"("Y"=w251, "X"=w222) -> ("X * Y"=w267:cdb[])  [unwired: 8 in, 1 out]
                n88 = call-poly <vilib>:"Convolution.vi"("Y"=w251, "X"=w239) -> ("X * Y"=w250:cdb[])  [unwired: 8 in, 1 out]
                n89 = Complex To Re/Im(x + iy=w239) -> (x=w253:dbl[], y=w252:dbl[])
                n90 = Array Subset(array=w222, index=0, length=w219) -> (w221:i16[])
                n91 = Absolute Value(x=w267) -> (abs(x)=w266:dbl[])
                n92 = Array Size(array=w239) -> (size(s)=w238:i32)
                n93 = Absolute Value(x=w250) -> (abs(x)=w249:dbl[])
                n94 = Complex To Re/Im(x + iy=w222) -> (x=w269:i16[], y=w268:i16[])
                n95 = Greater Than 0?(x=w238) -> (x > 0?=w236:bool)
                n96 = local read "dt"() -> (w223:dbl)
                n97 = Bundle By Name("dt"=w223, "Y"=w221) -> (w225:waveform(i16))  [unwired: 1 in]
                n98 = Array Max & Min(array=w266) -> (max index (indices)=w264:i32)  [unwired: 3 out]
                "max corr index" <- w264
                n99 = Array Size(array=w251) -> (size(s)=w247:i32)
                n100 = Build Array(w269, w268, w266, w253, w252, w249) -> (w271:dbl[][])
                n101 = Array Max & Min(array=w249) -> (max index (indices)=w248:i32)  [unwired: 3 out]
                n102 = To Single Precision Float(number=w271) -> (single precision float=w229:sgl[][])
                n103 = Subtract(x=w264, y=w247) -> (x-y=w263:i32)
                "compensated max" <- w263
                n104 = Subtract(x=w248, y=w247) -> (x-y=w245:i32)
                n105 = local read "dt"() -> (w244:dbl)
                n106 = To Double Precision Float(number=w263) -> (double precision float=w262:dbl)
                n107 = To Double Precision Float(number=w245) -> (double precision float=w246:dbl)
                n108 = case shown="True" "Plot" {
                  tunnel: w229 -> [_ w280]
                  frame False {
                  }
                  frame True {
                    "Waveform plot" <- w280
                  }
                }
                n109 = Multiply(x=w244, y=w262) -> (x*y=w235:dbl)
                "RXA-TX delay" <- w235
                n110 = Multiply(x=w244, y=w246) -> (x*y=w234:dbl)
                "RXB-TX delay" <- w234
                n111 = call-poly <vilib>:"FFT Power Spectrum and PSD.vi"("export mode"=w226, "averaging parameters"="averaging parameters", "restart averaging (F)"="Averaging control", "dB On (F)"=TRUE, "window"=w228, "time signal"=w225) -> ("Power Spectrum / PSD"=→"Power spectrum":cluster{"f0":dbl, "df":dbl, "magnitude":dbl[]})  [unwired: 2 in, 3 out]
                n112 = Subtract(x=w235, y=w234) -> (x-y=w233:dbl)
                n113 = case shown="True" w236 {
                  tunnel: "Reset statistics" -> [_ w279]
                  tunnel: w234 -> [_ w278]
                  tunnel: [_ w277] -> w241
                  tunnel: [_ w276] -> w237
                  tunnel: w233 -> [_ w275]
                  tunnel: "Reset statistics" -> [_ w274]
                  tunnel: [_ w273] -> w231
                  tunnel: [_ w272] -> w230
                  frame False {
                  }
                  frame True {
                    n114 = call "Statistics calculation real-time C.vi"("Reset calc"=w274, "new data"=w275) -> ("Statistics"=w272:cluster{"Count":i32, "Mean":dbl, "Std":dbl}, "Histogram Graph"=w273:T44)  [unwired: 8 in]
                    n115 = call "Statistics calculation real-time B.vi"("Reset calc"=w279, "new data"=w278) -> ("Statistics"=w276:cluster{"Count":i32, "Mean":dbl, "Std":dbl}, "Histogram Graph"=w277:T44)  [unwired: 8 in]
                  }
                }
                "RXB-TXA stat" <- w237
                "RXB-RXA stat" <- w230
                n116 = call "Statistics calculation real-time A.vi"("Reset calc"="Reset statistics", "new data"=w235) -> ("Statistics"=→"RXA-TXA stat":cluster{"Count":i32, "Mean":dbl, "Std":dbl}, "Histogram Graph"=w243:T44)  [unwired: 8 in]
                n117 = Build Array(w243, w241, w231) -> (→"Time histogram":T3)
              }
            }
          }
          frame "txrx.trig" {
            n118 = for {
              tunnel: w284 -> [w295] mode=indexing
              tunnel: [w293] -> w282 mode=indexing
              n119 = Unbundle By Name(w295) -> ("hardware configuration.direction"=w292:T25, "tx baseband session.7902 reference"=w294:T37)
              n120 = case shown="\"Transceiver\", \"Transmitter\"" w292 {
                tunnel: w294 -> [w303 _]
                tunnel: [w301 _] -> w293
                frame "Transceiver", "Transmitter" {
                  w298 = u64 1000000000000  # repeat
                  w299 = u64 1  # repeat
                  n121 = local read "last wr addr"() -> (w302:u32)
                  n122 = Select(t=w298, s="Repeat", f=w299) -> (s? t:f=w297:u64)
                  n123 = Bundle By Name(cluster=T26 {"start addr"=0, "end addr"=299, "repeat"=1} ("seq.new step"), "end addr"=w302, "repeat"=w297) -> (w307:T26)
                  n124 = call "SEQ Reset sequencer.vi"("Refnum in"=w303) -> ("error out"=w308:errorcluster, "Refnum out"=w309:T45)  [unwired: 9 in]
                  n125 = call "SEQ Add sequence step.vi"("error in (no error)"=w308, "seq.new step"=w307, "Refnum in"=w309) -> ("error out"=w306:errorcluster, "Refnum out"=w305:T45)  [unwired: 7 in]
                  n126 = call "SEQ Start sequence.vi"("error in (no error)"=w306, "sequence.cont"=FALSE, "Refnum in"=w305) -> ("error out"=w301:errorcluster)  [unwired: 7 in, 1 out]
                }
                frame "Receiver" {
                }
              }
            }
            n127 = Enqueue Element(queue=w288, element=T21 {"message"="txrx.fetch", "data"=variant}) -> ()  [unwired: 2 in, 3 out]
            n128 = Merge Errors(w282) -> (w281:errorcluster)
            n129 = call "Send Sync Trigger.vi"("session in"=w284, "sync select"=Direction."Transceiver", "master device index"=0, "error in"=w281) -> ("session out"=w289:T29[], "error out"=w283:errorcluster)  [unwired: 10 in]
          }
          frame "txrx.stop" {
            # "#todo\nmake stop driver functions"
          }
        }
        n130 = local write "State"(w190) -> ()
      }
      frame "exit" {
      }
    }
    "error out" <- w34
    n131 = call <vilib>:"Simple Error Handler.vi"("type of dialog (OK msg:1)"=w32, "error in (no error)"=w34) -> ()  [unwired: 3 in, 5 out]
  }
  n132 = while {
    tunnel: w8 -> [w320]
    tunnel: w9 -> [w317]
    tunnel: w5 -> [w316]
    stop <- w321 stop-if-true
    n133 = event shown="[9] \"SysB.Connect\": Value Change" {
      selector: _ -> [_ _ _ _ _ _ _ _ _ _ _ _ _]
      dyn-events: _ -> [_ _ _ _ _ _ _ _ _ _ _ _ _]
      timeout: 500 -> [_ _ _ _ _ _ _ _ _ _ _ _ _]
      tunnel: [_ TRUE _ _ _ _ _ _ _ _ _ _ _] -> w321
      tunnel: w320 -> [_ w330 w342 w374 w376 w397 _ w421 w425 _ _ _ _]
      tunnel: [_ _ _ _ _ w389 _ _ _ w433 w439 w444 w448] -> w319
      tunnel: w317 -> [w326 w332 _ _ _ _ _ _ _ w431 w437 w442 w447]
      tunnel: w316 -> [w327 w333 _ _ _ _ _ _ _ w432 w438 w443 w446]
      event Timeout {
        n134 = event-data() -> ()  [unwired: 1 in, 3 out]
        n135 = call-dynamic "Send Command.vi"("reference in"=w327, "message"="status", "error in (no error)"=w326, "response?"=TRUE) -> ("reponse"=→"Status":string, "error out"=w324:errorcluster)  [unwired: 7 in, 3 out]
        n136 = call <vilib>:"Clear Errors.vi"("error in (no error)"=w324) -> ()  [unwired: 5 in, 2 out]
      }
      event "Stop Button": Value Change {
        n137 = event-data() -> ()  [unwired: 1 in, 2 out]
        n138 = Enqueue Element(queue=w330, element=T21 {"message"="txrx.stop", "data"=variant}) -> (queue out=w328:refnum<queue>)  [unwired: 2 in, 2 out]
        n139 = Enqueue Element(queue=w328, element=T21 {"message"="exit", "data"=variant}) -> ()  [unwired: 2 in, 3 out]
        n140 = call-dynamic "Destroy.vi"("reference in"=w333, "error in (no error)"=w332) -> ("error out"=w334:errorcluster)  [unwired: 16 in, 1 out]
        n141 = local write "stop scirpt"(TRUE ("stop scirpt")) -> ()
        n142 = call <vilib>:"Clear Errors.vi"("error in (no error)"=w334) -> ()  [unwired: 5 in, 2 out]
      }
      event "hw.init": Value Change {
        n143 = event-data() -> ("CtlRef"=w337:refnum<vi>)  [unwired: 1 in]
        n144 = local read "TX trigger options"() -> (w343:T15)
        n145 = local read "RX trigger options"() -> (w351:T15)
        n146 = local read "RF config"() -> (w360:T14)
        n147 = local read "HW.trig share config"() -> (w352:T18)
        n148 = property class="Bool (strict)"(reference=w337, "Value"=FALSE) -> ()  [unwired: 1 in, 2 out]
        n149 = Build Array(w343, w351) -> (w344:T15[])
        n150 = Bundle By Name(cluster=T21 {"message"="hw.txrx init", "data"=variant} ("element"), "data"="HW.TXRX resources") -> (w363:T21)
        n151 = Bundle By Name(cluster=T21 {"message"="hw.txrx rf config", "data"=variant} ("element"), "data"=w360) -> (w358:T21)
        n152 = Bundle By Name(cluster=T21 {"message"="hw.txrx trig config", "data"=variant} ("element"), "data"=w344) -> (w356:T21)
        n153 = Bundle By Name(cluster=T21 {"message"="hw.trig share config", "data"=variant} ("element"), "data"=w352) -> (w353:T21)
        n154 = Enqueue Element(queue=w342, element=T21 {"message"="hw.close", "data"=variant}) -> (queue out=w341:refnum<queue>, error out=w340:errorcluster)  [unwired: 2 in, 1 out]
        n155 = Enqueue Element(queue=w341, element=w363, error in (no error)=w340) -> (queue out=w362:refnum<queue>, error out=w348:errorcluster)  [unwired: 1 in, 1 out]
        n156 = Enqueue Element(queue=w362, element=w358, error in (no error)=w348) -> (queue out=w359:refnum<queue>, error out=w347:errorcluster)  [unwired: 1 in, 1 out]
        n157 = Enqueue Element(queue=w359, element=w356, error in (no error)=w347) -> (queue out=w355:refnum<queue>, error out=w346:errorcluster)  [unwired: 1 in, 1 out]
        n158 = Enqueue Element(queue=w355, element=w353, error in (no error)=w346) -> (queue out=w350:refnum<queue>, error out=w345:errorcluster)  [unwired: 1 in, 1 out]
        n159 = Enqueue Element(queue=w350, element=T21 {"message"="ready", "data"=variant}, error in (no error)=w345) -> ()  [unwired: 1 in, 3 out]
      }
      event "hw.conf trig": Value Change {
        n160 = event-data() -> ()  [unwired: 1 in, 6 out]
        n161 = Build Array("TX trigger options", "RX trigger options") -> (w367:T15[])
        n162 = Bundle By Name(cluster=T21 {"message"="hw.txrx trig config", "data"=variant} ("element"), "data"=w367) -> (w371:T21)
        n163 = Bundle By Name(cluster=T21 {"message"="hw.trig share config", "data"=variant} ("element"), "data"="HW.trig share config") -> (w370:T21)
        n164 = Enqueue Element(queue=w374, element=w371) -> (queue out=w375:refnum<queue>)  [unwired: 2 in, 2 out]
        n165 = Enqueue Element(queue=w375, element=w370) -> ()  [unwired: 2 in, 3 out]
      }
      event Value Change {
        n166 = event-data() -> ()  [unwired: 1 in, 6 out]
        n167 = Bundle By Name(cluster=T21 {"message"="hw.txrx rf config", "data"=variant} ("element"), "data"="RF config") -> (w379:T21)
        n168 = Enqueue Element(queue=w376, element=w379) -> ()  [unwired: 2 in, 3 out]
      }
      event "txrx.start": Value Change {
        n169 = event-data() -> ("CtlRef"=w393:refnum<vi>)  [unwired: 1 in, 1 out]
        n170 = String To Path(string="IQ waveform") -> (path=w385:path)
        n171 = Read from Binary File(5:cdb[] [] ("TX.IQ signal"), 11:w385) -> (0:w390:errorcluster, 2:w388:cdb[])  [unwired: 4 in, 2 out]
        n172 = Complex To Re/Im(x + iy=w388) -> (x=w384:dbl[], y=w383:dbl[])
        n173 = local read "dt"() -> (w380:dbl)
        n174 = Bundle By Name(cluster=T24 {"RX.read config"={"Samples"=16000}, "TX.IQ signal"=[1.0+0.0i], "TX.IQ Fs"=50000000.0, "TX burst/continuous"=TRUE, "TX.IQ samples"=1600} ("TXRX config"), "TX.IQ signal"=w388, "RX.read config"="RX.read config") -> (w394:T24)
        n175 = Bundle By Name("dt"=w380, "Y"=w384) -> (w381:waveform(dbl))  [unwired: 1 in]
        n176 = Bundle By Name(cluster=w381, "Y"=w383) -> (w382:waveform(dbl))
        n177 = property class="Bool (strict)"(reference=w393, "Value"=FALSE) -> ()  [unwired: 1 in, 2 out]
        n178 = Build Array(w381, w382) -> (→"IQ preview":waveform(dbl)[])
        n179 = Bundle By Name(cluster=T21 {"message"="txrx.start", "data"=variant} ("element"), "data"=w394) -> (w398:T21)
        n180 = Enqueue Element(queue=w397, element=w398, error in (no error)=w390) -> (error out=w389:errorcluster)  [unwired: 1 in, 2 out]
      }
      event "IQ waveform": Value Change {
        w401 = 64 ("x")
        n181 = event-data() -> ("NewVal"=w416:string)  [unwired: 1 in, 5 out]
        n182 = String To Path(string=w416) -> (path=w415:path)
        n183 = Read from Binary File(5:cdb[] [] ("TX.IQ signal"), 11:w415) -> (2:w402:cdb[])  [unwired: 4 in, 3 out]
        n184 = Array Size(array=w402) -> (size(s)=w408:i32)
        n185 = Quotient & Remainder(x=w408, y=w401) -> (x-y*floor(x/y)=w407:i32)  [unwired: 1 out]
        n186 = Subtract(x=w401, y=w407) -> (x-y=w404:i32)
        n187 = Quotient & Remainder(x=w404, y=w401) -> (x-y*floor(x/y)=w403:i32)  [unwired: 1 out]
        n188 = Initialize Array(cdb 0.0+0.0i ("element"), w403) -> (w406:cdb[])
        n189 = local read "dt"() -> (w410:dbl)
        n190 = Build Array (concatenate)(w402, w406) -> (w400:cdb[])
        n191 = Complex To Re/Im(x + iy=w400) -> (x=w414:dbl[], y=w413:dbl[])
        n192 = Bundle By Name("dt"=w410, "Y"=w414) -> (w411:waveform(dbl))  [unwired: 1 in]
        n193 = Bundle By Name(cluster=w411, "Y"=w413) -> (w412:waveform(dbl))
        n194 = Build Array(w411, w412) -> (w409:waveform(dbl)[])
        n195 = local write "IQ preview"(w409) -> ()
      }
      event "txrx.stop": Value Change {
        n196 = event-data() -> ("CtlRef"=w418:refnum<vi>)  [unwired: 1 in, 1 out]
        n197 = property class="Bool (strict)"(reference=w418, "Value"=FALSE) -> ()  [unwired: 1 in, 2 out]
        n198 = Enqueue Element(queue=w421, element=T21 {"message"="txrx.stop", "data"=variant}) -> ()  [unwired: 2 in, 3 out]
      }
      event "txrx.trigger": Value Change {
        n199 = event-data() -> ("CtlRef"=w422:refnum<vi>)  [unwired: 1 in, 1 out]
        n200 = property class="Bool (strict)"(reference=w422, "Value"=FALSE) -> ()  [unwired: 1 in, 2 out]
        n201 = Enqueue Element(queue=w425, element=T21 {"message"="txrx.trig", "data"=variant}) -> ()  [unwired: 2 in, 3 out]
      }
      event "SysB.Connect": Value Change {
        n202 = event-data() -> ()  [unwired: 1 in, 2 out]
        n203 = call-dynamic "Disconnect.vi"("error in (no error)"=w431, "reference in"=w432) -> ("error out"=w434:errorcluster, "reference out"=w428:refnum<class "NS master.lvclass">)  [unwired: 8 in]
        n204 = call <vilib>:"Clear Errors.vi"("error in (no error)"=w434) -> ()  [unwired: 5 in, 2 out]
        n205 = property class="NS master"(reference=w428, "properties:slave ip"="Sys B IP address", "properties:slave id"="SysB" ("Slave ID")) -> (reference out=w426:refnum<class "NS master.lvclass">, error out=w427:errorcluster)  [unwired: 1 in]
        n206 = call-dynamic "Connect.vi"("error in (no error)"=w427, "reference in"=w426) -> ("error out"=w433:errorcluster)  [unwired: 8 in, 1 out]
      }
      event "SysB.hw reinit": Value Change {
        n207 = event-data() -> ()  [unwired: 1 in, 6 out]
        n208 = flat-sequence {
          tunnel: w437 -> [w441]
          tunnel: [w441] -> w436
          frame #0 {
          }
        }
        n209 = call-dynamic "Send Command.vi"("reference in"=w438, "message"="hw.reinit", "error in (no error)"=w436, "response?"=FALSE) -> ("error out"=w439:errorcluster)  [unwired: 7 in, 4 out]
      }
      event "SysB.start rx": Value Change {
        n210 = event-data() -> ()  [unwired: 1 in, 6 out]
        n211 = call-dynamic "Send Command.vi"("reference in"=w443, "message"="rx.start", "error in (no error)"=w442) -> ("error out"=w444:errorcluster)  [unwired: 8 in, 4 out]
      }
      event "SysB.stop rx": Value Change {
        n212 = event-data() -> ()  [unwired: 1 in, 6 out]
        n213 = call-dynamic "Send Command.vi"("reference in"=w446, "message"="rx.stop", "error in (no error)"=w447) -> ("error out"=w448:errorcluster)  [unwired: 8 in, 4 out]
      }
    }
    n214 = call <vilib>:"Simple Error Handler.vi"("error in (no error)"=w319) -> ()  [unwired: 4 in, 5 out]
  }
  n215 = while {
    tunnel: w8 -> [_]
    tunnel: w6 -> [w451]
    tunnel: w5 -> [w450]
    stop <- "stop scirpt" stop-if-true
    # "Script execution"
    n216 = case shown="True" "Script.start" {
      tunnel: "Script" -> [_ w465]
      tunnel: w451 -> [_ w458]
      tunnel: w450 -> [_ w457]
      frame False {
        n217 = Wait (ms)(milliseconds to wait=u32 1) -> ()  [unwired: 1 out]
      }
      frame True {
        n218 = call <vilib>:"Trim Whitespace.vi"("string"=w465) -> ("trimmed string"=w460:string)  [unwired: 1 in]
        n219 = Spreadsheet String To Array(delimiter (Tab)="\n", format string="%s", spreadsheet string=w460, array type (2D Dbl)=string[] []) -> (array=w461:string[])
        n220 = for {
          tunnel: w461 -> [w520] mode=indexing
          tunnel: [w497] -> w459 mode=indexing
          n221 = Match Pattern(string=w520, regular expression="\"") -> (before substring=w516:string, after substring=w517:string)  [unwired: 1 in, 2 out]
          n222 = Match Pattern(string=w517, regular expression="\"") -> (before substring=w515:string, after substring=w509:string)  [unwired: 1 in, 2 out]
          n223 = Match Pattern(string=w509, regular expression="D") -> (after substring=w513:string)  [unwired: 1 in, 3 out]
          n224 = Match Pattern(string=w509, regular expression="R") -> (after substring=w500:string)  [unwired: 1 in, 3 out]
          n225 = call <vilib>:"Trim Whitespace.vi"("string"=w516) -> ("trimmed string"=w506:string)  [unwired: 1 in]
          n226 = call <vilib>:"Trim Whitespace.vi"("string"=w515) -> ("trimmed string"=w505:string)  [unwired: 1 in]
          n227 = call <vilib>:"Trim Whitespace.vi"("string"=w513) -> ("trimmed string"=w512:string)  [unwired: 1 in]
          n228 = call <vilib>:"Trim Whitespace.vi"("string"=w500) -> ("trimmed string"=w501:string)  [unwired: 1 in]
          n229 = Scan From String(format string="%d", input string=w512, default 1=0 ("default value 1")) -> (error out=w499:errorcluster, output 1=w504:i32)  [unwired: 2 in, 2 out]
          n230 = Scan From String(format string="%d", input string=w501, default 1=1 ("default value 1")) -> (error out=w496:errorcluster, output 1=w498:i32)  [unwired: 2 in, 2 out]
          n231 = Bundle By Name(cluster=T4 {"System"="", "Command"="", "Delay"=0, "Repeat"=0} ("Command"), "System"=w506, "Command"=w505, "Delay"=w504, "Repeat"=w498) -> (w497:T4)
          n232 = call <vilib>:"Clear Errors.vi"("error in (no error)"=w496) -> ()  [unwired: 5 in, 2 out]
          n233 = call <vilib>:"Clear Errors.vi"("error in (no error)"=w499) -> ()  [unwired: 5 in, 2 out]
        }
        n234 = for {
          N: "Repeat script" -> [_]
          tunnel: w459 -> [w469]
          tunnel: w458 -> [w468]
          tunnel: w457 -> [w467]
          i -> [w466]
          n235 = for {
            tunnel: w469 -> [w477] mode=indexing
            tunnel: w468 -> [w474]
            tunnel: w467 -> [w471]
            i -> [w470]
            n236 = Unbundle By Name(w477) -> ("Repeat"=w476:i32, "System"=w475:string, "Command"=w473:string, "Delay"=w472:i32)
            n237 = for {
              N: w476 -> [_]
              tunnel: w475 -> [w484]
              tunnel: w474 -> [w483]
              tunnel: w473 -> [w482]
              tunnel: w472 -> [w480]
              tunnel: w471 -> [w479]
              i -> [w478]
              n238 = case shown="\"A\", Default" w484 {
                tunnel: w483 -> [w489 _]
                tunnel: w482 -> [w488 w494]
                tunnel: ["" _] -> w481
                tunnel: w479 -> [_ w495]
                frame "A", Default {
                  n239 = Look In Map(map=w489, key=w488) -> (key not found?=w486:bool, value=w487:refnum<vi>)  [unwired: 1 in]
                  n240 = case shown="False" w486 {
                    tunnel: w487 -> [w492 w493]
                    tunnel: [w490 w493] -> _
                    frame False {
                      n241 = property class="Ctl"(reference=w492, "Val(Sgnl)"=TRUE) -> (reference out=w490:refnum<vi>)  [unwired: 1 in, 1 out]
                    }
                    frame True {
                    }
                  }
                }
                frame "B" {
                  n242 = call-dynamic "Send Command.vi"("reference in"=w495, "message"=w494) -> ()  [unwired: 9 in, 5 out]
                }
              }
              n243 = call "Stall Data Flow.vim"("value in"=w481, "milliseconds to wait"=w480) -> ()  [unwired: 2 out]
              "R ctr" <- w478
            }
            "Last executed command" <- w477
            "step ctr" <- w470
          }
          "script ctr" <- w466
        }
      }
    }
  }
  n244 = disable-structure shown="Disabled" {
    frame Disabled {
      n245 = flat-sequence {
        frame #0 {
          # "8"
          # "7"
          n246 = call <instrlib>:"niSync Disconnect Trigger Terminals.vi"() -> ("error out"=w523:errorcluster, "instrument handle out"=w522:refnum<k15>)  [unwired: 10 in]
          n247 = call <instrlib>:"niSync Close.vi"("error in (no error)"=w523, "instrument handle"=w522) -> ("error out"=w521:errorcluster)  [unwired: 9 in]
          n248 = call <vilib>:"Clear Errors.vi"("error in (no error)"=w521) -> ()  [unwired: 5 in, 2 out]
        }
      }
    }
    frame Enabled {
    }
  }
